vi "ReadPropertiesStatesCommandsH.vi"() -> ()   [LabVIEW 2010]
panel:
  in  "ShutterButton":u32(ring) items=["_OFF"=0, "_Halfway"=1, "_Completely"=3, "_Halfway_NonAF"=65537, "_Completely_NonAF"=65539]
  in  "kEdsCameraStatusCommand":u32(ring) items=["UILock", "UIUnLock", "EnterDirectTransfer", "ExitDirectTransfer"]
  in  "kEdsImageTypes":u32(ring) items=["Unknown"=0, "Jpeg"=1, "CRW"=2, "RAW"=4, "CR2"=6, "MOVwithTHM"=12, "MOVwithoutTHM"=13]
  in  "kEdsWhiteBalance":i32(ring) items=["Auto"=0, "Daylight"=1, "Cloudy"=2, "Tangsten"=3, "Fluorescent"=4, "Strobe"=5, "WhitePaper"=6, "Shade"=8, "ColorTemp"=9, "PCSet1"=10, "PCSet2"=11, "PCSet3"=12, "WhitePaper2"=15, "WhitePaper3"=16, "WhitePaper4"=18, "WhitePaper5"=19, "PCSet4"=20, "PCSet5"=21, "Click"=-1, "Pasted"=-2]
  in  "EdsImageQuality":u32(ring) items=["LJ"=1113871, "M1J"=84999951, "M2J"=101777167, "SJ"=34668303, "LJF"=1310479, "LJN"=1244943, "MJF"=18087695, "MJN"=18022159, "SJF"=34864911, "SJN"=34799375, "S1JF"=236191503, "S1JN"=236125967, "S2JF"=252968719, "S3JF"=269745935, "LR"=6618895, "LRLJF"=6553619, "LRLJN"=6553618, "LRMJF"=6553875, "LRMJN"=6553874, "LRSJF"=6554131, "LRSJN"=6554130, "LRS1JF"=6557203, "LRS1JN"=6557202, "LRS2JF"=6557459, "LRS3JF"=6557715, "LRLJ"=6553616, "LRM1J"=6554896, "LRM2J"=6555152, "LRSJ"=6554128, "MR"=23396111, "MRLJF"=23330835, "MRLJN"=23330834, "MRMJF"=23331091, "MRMJN"=23331090, "MRSJF"=23331347, "MRSJN"=23331346, "MRS1JF"=23334419, "MRS1JN"=23334418, "MRS2JF"=23334675, "MRS3JF"=23334931, "MRLJ"=23330832, "MRM1J"=23332112, "MRM2J"=23332368, "MRSJ"=23331344, "SR"=40173327, "SRLJF"=40108051, "SRLJN"=40108050, "SRMJF"=40108307, "SRMJN"=40108306, "SRSJF"=40108563, "SRSJN"=40108562, "SRS1JF"=40111635, "SRS1JN"=40111634, "SRS2JF"=40111891, "SRS3JF"=40112147, "SRLJ"=40108048, "SRM1J"=40109328, "SRM2J"=40109584, "SRSJ"=40108560, "Unknown"=4294967295]
  in  "kEdsAEMode":u32(ring) items=["Program"=0, "Tv"=1, "Av"=2, "Manual"=3, "Bulb"=4, "A_DEP"=5, "DEP"=6, "Custom"=7, "Lock"=8, "Green"=9, "NightPortrait"=10, "Sports"=11, "Portrait"=12, "Landscape"=13, "Closeup"=14, "FlashOff"=15, "CreativeAuto"=19, "Movie"=20, "PhotoInMovie"=21, "Unknown"=4294967295]
  in  "kEdsStorageType":u32(ring) items=["Non"=0, "CF"=1, "SD"=2, "HD"=4]
  in  "kEdsTargetImageTypes":u32(ring) items=["Unknown"=0, "Jpeg"=1, "TIFF"=7, "TIFF16"=8, "RGB"=9, "RGB16"=10, "DIB"=11]
  in  "kEdsDataTypes":u32(ring) items=["Unknown"=0, "Bool"=1, "String"=2, "Int8"=3, "UInt8"=6, "Int16"=4, "UInt16"=7, "Int32"=8, "UInt32"=9, "Int64"=10, "UInt64"=11, "Float"=12, "Double"=13, "ByteBlock"=14, "Rational"=20, "Point"=21, "Rect"=22, "Time"=23, "Bool_Array"=30, "Int8_Array"=31, "Int16_Array"=32, "Int32_Array"=33, "UInt8_Array"=34, "UInt16_Array"=35, "UInt32_Array"=36, "Rational_Array"=37, "FocusInfo"=101]
  in  "kEdsStateEvents":u32(ring) items=["All"=768, "Shutdown"=769, "JobStatusChanged"=770, "WillSoonShutDown"=771, "ShutDownTimerUpdate"=772, "CaptureError"=773, "InternalError"=774, "AfResult"=777, "BulbExposureTime"=784]
  in  "kEdsObjectEvents":u32(ring)=512 items=["All"=512, "VolumeInfoChanged"=513, "VolumeUpdateItems"=514, "FolderUpdateItems"=515, "DirItemCreated"=516, "DirItemRemoved"=517, "DirItemInfoChanged"=518, "DirItemContentChanged"=519, "DirItemRequestTransfer"=520, "DirItemRequestTransferDT"=521, "DirItemCancelTransferDT"=522, "VolumeAdded"=524, "VolumeRemoved"=525]
  in  "kEdsPropertyEvents":u32(ring) items=["All"=256, "PropertyChanged"=257, "PropertyDescChanged"=258]
  in  "kEdsCameraCommands":u32(ring) items=["TakePicture"=0, "ExtendShutDownTimer"=1, "BulbStart"=2, "BulbEnd"=3, "DoEvfAf"=258, "DriveLensEvf"=259, "DoClickWBEvf"=260, "PressShutterButton"=4]
  in  "kEdsPropIDs":u32(ring) items=["Unknown"=65535, "ProductName"=2, "BodyID"=3, "OwnerName"=4, "MakerName"=5, "DateTime"=6, "FirmwareVersion"=7, "BatteryLevel"=8, "CFn"=9, "SaveTo"=11, "CurrentStorage"=12, "CurrentFolder"=13, "MyMenu"=14, "BatteryQuality"=16, "HDDirectoryStructure"=32, "ImageQuality"=256, "JpegQuality"=257, "Orientation"=258, "ICCProfile"=259, "FocusInfo"=260, "DigitalExposure"=261, "WhiteBalance"=262, "ColorTemperature"=263, "WhiteBalanceShift"=264, "Contrast"=265, "ColorSaturation"=266, "ColorTone"=267, "Sharpness"=268, "ColorSpace"=269, "ToneCurve"=270, "PhotoEffect"=271, "FilterEffect"=272, "ToningEffect"=273, "ParameterSet"=274, "ColorMatrix"=275, "PictureStyle"=276, "PictureStyleDesc"=277, "ETTL2Mode"=279, "PictureStyleCaption"=512, "Linear"=768, "ClickWBPoint"=769, "WBCoeffs"=770, "GPSVersionID"=2048, "GPSLatitudeRef"=2049, "GPSLatitude"=2050, "GPSLongitudeRef"=2051, "GPSLongitude"=2052, "GPSAltitudeRef"=2053, "GPSAltitude"=2054, "GPSTimeStamp"=2055, "GPSSatellites"=2056, "GPSStatus"=2057, "GPSMapDatum"=2066, "GPSDateStamp"=2077, "AtCapture_Flag"=2147483648, "AEMode"=1024, "DriveMode"=1025, "ISOSpeed"=1026, "MeteringMode"=1027, "AFMode"=1028, "Av"=1029, "Tv"=1030, "ExposureCompensation"=1031, "FlashCompensation"=1032, "FocalLength"=1033, "AvailableShots"=1034, "Bracket"=1035, "WhiteBalanceBracket"=1036, "LensName"=1037, "AEBracket"=1038, "FEBracket"=1039, "ISOBracket"=1040, "NoiseReduction"=1041, "FlashOn"=1042, "RedEye"=1043, "FlashMode"=1044, "LensStatus"=1046, "Artist"=1048, "Copyright"=1049, "DepthOfField"=1051, "EFCompensation"=1054, "Evf_OutputDevice"=1280, "Evf_Mode"=1281, "Evf_WhiteBalance"=1282, "Evf_ColorTemperature"=1283, "Evf_DepthOfFieldPreview"=1284, "Evf_Zoom"=1287, "Evf_ZoomPosition"=1288, "Evf_FocusAid"=1289, "Evf_Histogram"=1290, "Evf_ImagePosition"=1291, "Evf_HistogramStatus"=1292, "Evf_AFMode"=1294, "Evf_CoordinateSystem"=1344, "Evf_ZoomRect"=1345]
  # "Copy-paste these controls as type definitions\nor \"customize\" them to save them in the library\nas type defs"
  # "#define"
  # "#enum"
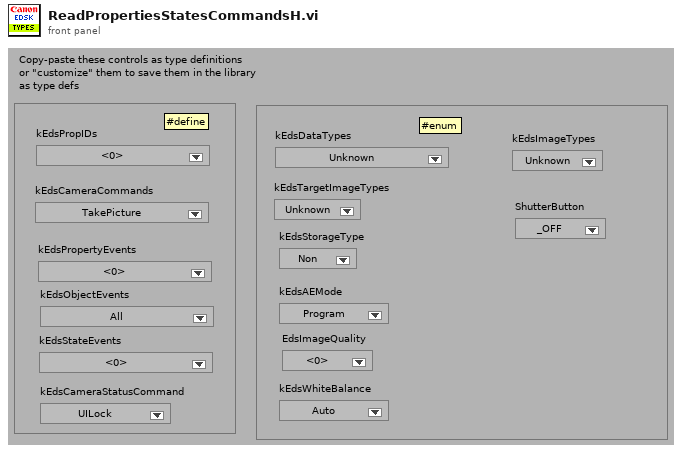
[diagram p1: front panel]
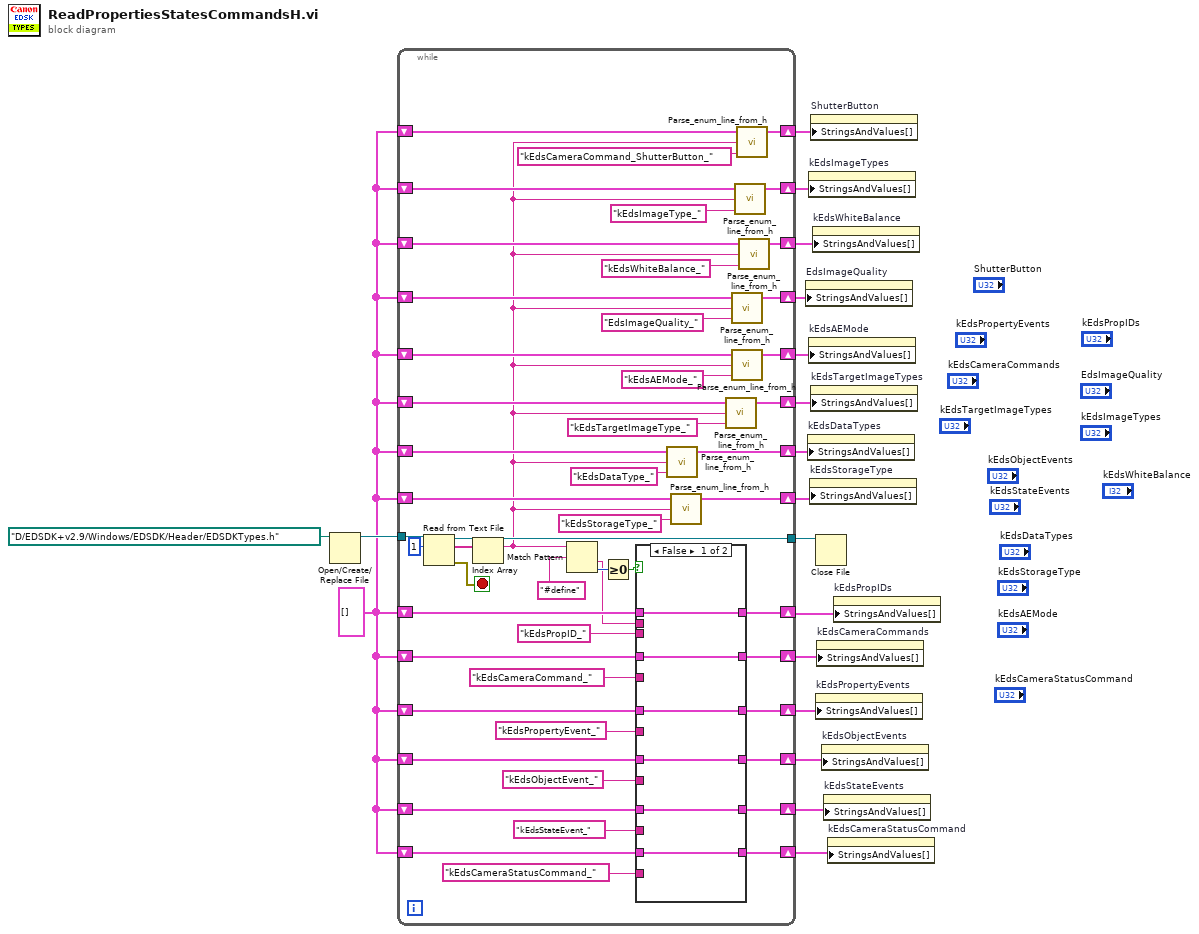
[diagram p0: block diagram]
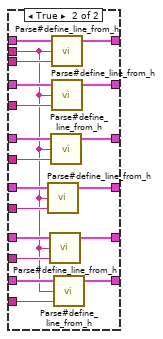
[diagram p2: hidden frame]
diagram:
  w1 = cluster{string, u32}[] []
  n1 = Open/Create/Replace File(file path (use dialog)=path "D:/EDSDK+v2.9/Windows/EDSDK/Header/EDSDKTypes.h") -> (refnum out=w17:refnum<file>)  [unwired: 5 in, 2 out]
  n2 = while {
    tunnel: w17 -> [w70]
    tunnel: [w61] -> w16
    shift-right: [w64] -> w15
    shift-left: w1 -> [w65]
    shift-right: [w57] -> w14
    shift-left: w1 -> [w58]
    shift-right: [w54] -> w13
    shift-left: w1 -> [w55]
    shift-right: [w50] -> w12
    shift-left: w1 -> [w51]
    shift-right: [w49] -> w11
    shift-left: w1 -> [w48]
    shift-right: [w44] -> w10
    shift-left: w1 -> [w46]
    shift-right: [w43] -> w9
    shift-left: w1 -> [w41]
    shift-right: [w38] -> w8
    shift-left: w1 -> [w39]
    shift-right: [w35] -> w7
    shift-left: w1 -> [w37]
    shift-right: [w34] -> w6
    shift-left: w1 -> [w32]
    shift-right: [w30] -> w5
    shift-left: w1 -> [w31]
    shift-right: [w27] -> w4
    shift-left: w1 -> [w26]
    shift-right: [w23] -> w3
    shift-left: w1 -> [w24]
    shift-right: [w21] -> w2
    shift-left: w1 -> [w22]
    stop <- w68 stop-if-true
    n3 = Read from Text File(file (use dialog)=w70, count=1) -> (refnum out=w61:refnum<file>, text=w62:string[], error out=w68:errorcluster)  [unwired: 2 in, 1 out]
    n4 = Index Array(array=w62) -> (element=w19:string)  [unwired: 1 in]
    n5 = Match Pattern(string=w19, regular expression="#define") -> (after substring=w59:string, offset past match=w67:i32)  [unwired: 1 in, 2 out]
    n6 = Greater Or Equal To 0?(x=w67) -> (x >= 0?=w66:bool)
    n7 = case shown="False" w66 {
      tunnel: w65 -> [w76 w92]
      tunnel: [w76 w90] -> w64
      tunnel: w59 -> [_ w77]
      tunnel: "kEdsPropID_" ("regular expression") -> [_ w91]
      tunnel: w58 -> [w75 w95]
      tunnel: [w75 w94] -> w57
      tunnel: "kEdsCameraCommand_" ("regular expression") -> [_ w93]
      tunnel: w55 -> [w74 w89]
      tunnel: [w74 w88] -> w54
      tunnel: "kEdsPropertyEvent_" ("regular expression") -> [_ w87]
      tunnel: w51 -> [w73 w84]
      tunnel: [w73 w85] -> w50
      tunnel: "kEdsObjectEvent_" ("regular expression") -> [_ w86]
      tunnel: w48 -> [w72 w83]
      tunnel: [w72 w82] -> w49
      tunnel: "kEdsStateEvent_" ("regular expression") -> [_ w81]
      tunnel: w24 -> [w71 w78]
      tunnel: [w71 w79] -> w23
      tunnel: "kEdsCameraStatusCommand_" ("regular expression") -> [_ w80]
      frame False {
      }
      frame True {
        n8 = call "Parse#define_line_from_h.vi"("define prefix"=w86, "enum line"=w77, "define-values in"=w84) -> ("define-values out"=w85:cluster{string, u32}[])  [unwired: 2 in]
        n9 = call "Parse#define_line_from_h.vi"("define prefix"=w81, "enum line"=w77, "define-values in"=w83) -> ("define-values out"=w82:cluster{string, u32}[])  [unwired: 2 in]
        n10 = call "Parse#define_line_from_h.vi"("define prefix"=w87, "enum line"=w77, "define-values in"=w89) -> ("define-values out"=w88:cluster{string, u32}[])  [unwired: 2 in]
        n11 = call "Parse#define_line_from_h.vi"("define prefix"=w91, "enum line"=w77, "define-values in"=w92) -> ("define-values out"=w90:cluster{string, u32}[])  [unwired: 2 in]
        n12 = call "Parse#define_line_from_h.vi"("define prefix"=w93, "enum line"=w77, "define-values in"=w95) -> ("define-values out"=w94:cluster{string, u32}[])  [unwired: 2 in]
        n13 = call "Parse#define_line_from_h.vi"("define prefix"=w80, "enum line"=w77, "define-values in"=w78) -> ("define-values out"=w79:cluster{string, u32}[])  [unwired: 2 in]
      }
    }
    n14 = call "Parse_enum_line_from_h.vi"("enum prefix"="kEdsDataType_" ("define prefix"), "enum line"=w19, "enum-values in"=w46) -> ("enum-values out"=w44:cluster{string, i64}[])  [unwired: 2 in]
    n15 = call "Parse_enum_line_from_h.vi"("enum prefix"="kEdsStorageType_" ("define prefix"), "enum line"=w19, "enum-values in"=w39) -> ("enum-values out"=w38:cluster{string, i64}[])  [unwired: 2 in]
    n16 = call "Parse_enum_line_from_h.vi"("enum prefix"="kEdsTargetImageType_" ("define prefix"), "enum line"=w19, "enum-values in"=w41) -> ("enum-values out"=w43:cluster{string, i64}[])  [unwired: 2 in]
    n17 = call "Parse_enum_line_from_h.vi"("enum prefix"="EdsImageQuality_" ("define prefix"), "enum line"=w19, "enum-values in"=w32) -> ("enum-values out"=w34:cluster{string, i64}[])  [unwired: 2 in]
    n18 = call "Parse_enum_line_from_h.vi"("enum prefix"="kEdsAEMode_" ("define prefix"), "enum line"=w19, "enum-values in"=w37) -> ("enum-values out"=w35:cluster{string, i64}[])  [unwired: 2 in]
    n19 = call "Parse_enum_line_from_h.vi"("enum prefix"="kEdsImageType_" ("define prefix"), "enum line"=w19, "enum-values in"=w26) -> ("enum-values out"=w27:cluster{string, i64}[])  [unwired: 2 in]
    n20 = call "Parse_enum_line_from_h.vi"("enum prefix"="kEdsCameraCommand_ShutterButton_" ("define prefix"), "enum line"=w19, "enum-values in"=w22) -> ("enum-values out"=w21:cluster{string, i64}[])  [unwired: 2 in]
    n21 = call "Parse_enum_line_from_h.vi"("enum prefix"="kEdsWhiteBalance_" ("define prefix"), "enum line"=w19, "enum-values in"=w31) -> ("enum-values out"=w30:cluster{string, i64}[])  [unwired: 2 in]
  }
  n22 = property on="EdsImageQuality" class="Ring (strict)"("StringsAndValues[]"=w6) -> ()  [unwired: 2 in, 2 out]
  n23 = property on="kEdsDataTypes" class="Ring (strict)"("StringsAndValues[]"=w10) -> ()  [unwired: 2 in, 2 out]
  n24 = property on="kEdsImageTypes" class="Ring (strict)"("StringsAndValues[]"=w4) -> ()  [unwired: 2 in, 2 out]
  n25 = property on="kEdsAEMode" class="Ring (strict)"("StringsAndValues[]"=w7) -> ()  [unwired: 2 in, 2 out]
  n26 = property on="kEdsStorageType" class="Ring (strict)"("StringsAndValues[]"=w8) -> ()  [unwired: 2 in, 2 out]
  n27 = property on="ShutterButton" class="Ring (strict)"("StringsAndValues[]"=w2) -> ()  [unwired: 2 in, 2 out]
  n28 = property on="kEdsTargetImageTypes" class="Ring (strict)"("StringsAndValues[]"=w9) -> ()  [unwired: 2 in, 2 out]
  n29 = property on="kEdsWhiteBalance" class="Ring (strict)"("StringsAndValues[]"=w5) -> ()  [unwired: 2 in, 2 out]
  n30 = Close File(refnum=w16) -> ()  [unwired: 1 in, 2 out]
  n31 = property on="kEdsPropertyEvents" class="Ring (strict)"("StringsAndValues[]"=w13) -> ()  [unwired: 2 in, 2 out]
  n32 = property on="kEdsCameraCommands" class="Ring (strict)"("StringsAndValues[]"=w14) -> ()  [unwired: 2 in, 2 out]
  n33 = property on="kEdsObjectEvents" class="Ring (strict)"("StringsAndValues[]"=w12) -> ()  [unwired: 2 in, 2 out]
  n34 = property on="kEdsStateEvents" class="Ring (strict)"("StringsAndValues[]"=w11) -> ()  [unwired: 2 in, 2 out]
  n35 = property on="kEdsCameraStatusCommand" class="Ring (strict)"("StringsAndValues[]"=w3) -> ()  [unwired: 2 in, 2 out]
  n36 = property on="kEdsPropIDs" class="Ring (strict)"("StringsAndValues[]"=w15) -> ()  [unwired: 2 in, 2 out]
